vi "9239_2 - 副本.vi"() -> ()   [LabVIEW 2014]
panel:
  in  "路径":path
  out "采样频率":dbl
  in  "采样数":dbl=200.0
  in  "数据采集开关":bool
  out "已采样数量":dbl
  in  "采样率":dbl=2000.0
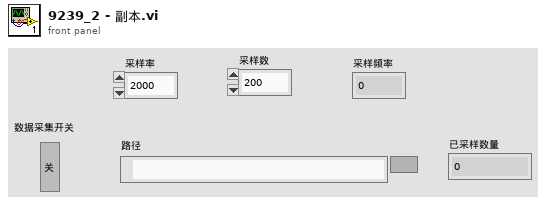
[diagram p1: front panel]
types:
  T1 = enum16{"open", "open or create", "create or replace", "create", "open (read-only)"}
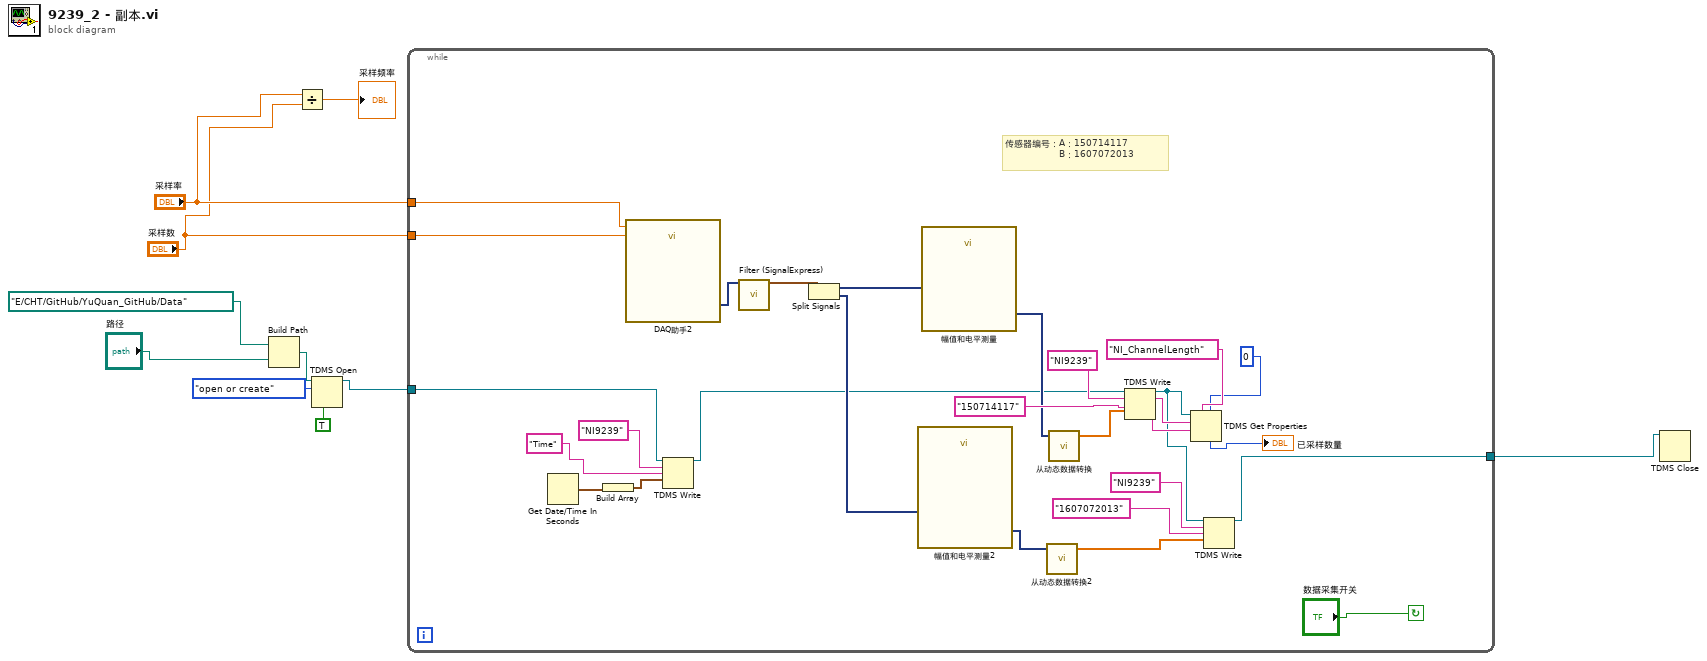
[diagram p0: block diagram]
diagram:
  n1 = Build Path(base path=path "E:/CHT/GitHub/YuQuan_GitHub/Data", name or relative path="路径") -> (appended path=w9:path)
  n2 = Divide(x="采样率", y="采样数") -> (x/y=→"采样频率":dbl)
  n3 = TDMS Open(6:TRUE ("disable buffering (T)"), 10:T1."open or create" ("operation"), 11:w9) -> (3:w5:refnum<k34>)  [unwired: 4 in, 1 out]
  n4 = while {
    tunnel: w5 -> [w16]
    tunnel: [w13] -> w4
    tunnel: "采样率" -> [w12]
    tunnel: "采样数" -> [w11]
    stop <- "数据采集开关" continue-if-true
    # "传感器编号：A：150714117\n                  B：1607072013"
    n5 = Get Date/Time In Seconds() -> (seconds since 1Jan1904=w20:timestamp)
    n6 = Build Array(w20) -> (w19:timestamp[])
    n7 = call "DAQ助手2"("速率"=w12, "采样数"=w11) -> ("data"=w38:dynamicdata)  [unwired: 14 in, 3 out]
    n8 = TDMS Write(0:w16, 5:"NI9239", 7:"Time", 9:w19) -> (4:w15:refnum<k34>)  [unwired: 2 in, 3 out]
    n9 = call "Filter (SignalExpress)"("input signals"=w38) -> ("filtered data"=w37:waveform(dbl)[])  [unwired: 17 in, 1 out]
    n10 = Split Signals(w37) -> (w23:dynamicdata, w22:dynamicdata)  [unwired: 2 in]
    n11 = call "幅值和电平测量2"("Signals"=w22) -> ("Mean (DC)"=w26:dynamicdata)  [unwired: 13 in, 1 out]
    n12 = call "幅值和电平测量"("Signals"=w23) -> ("Mean (DC)"=w34:dynamicdata)  [unwired: 13 in, 1 out]
    n13 = call "从动态数据转换2"("Dynamic Data Type"=w26) -> ("Array"=w24:dbl[])  [unwired: 3 in]
    n14 = call "从动态数据转换"("Dynamic Data Type"=w34) -> ("Array"=w25:dbl[])  [unwired: 3 in]
    n15 = TDMS Write(0:w15, 5:"NI9239", 7:"150714117", 9:w25) -> (4:w14:refnum<k34>, 6:w33:string, 8:w32:string)  [unwired: 2 in, 1 out]
    n16 = TDMS Get Properties(5:0, 7:"NI_ChannelLength", 9:w32, 10:w33, 11:w14) -> (4:→"已采样数量":i32)  [unwired: 1 in, 5 out]
    n17 = TDMS Write(0:w14, 5:"NI9239", 7:"1607072013", 9:w24) -> (4:w13:refnum<k34>)  [unwired: 2 in, 3 out]
  }
  n18 = TDMS Close(11:w4) -> ()  [unwired: 1 in, 2 out]
